vi "HEWH RLT PRAT.vi"() -> ()   [LabVIEW 2023] (continued)
            w3292 = 42 items=["No error", "Argument error", "Memory is full", "Out of zone", "End of file", "File already open", "Generic file I/O error", "File not found", "File permission error", "Disk is full", "Duplicate path", "Too many files open", "System feature not enabled", "Resource file not found", "Cannot add resource", "Resource not found", "Image not found", "Image memory error", "Pen does not exist", "Config type invalid", "Config token not found", "Config parse error", "Config memory error", "Bad external code format", "Bad external code offset", "External code not present", "Null window", "Destroy window error", "Null menu", "Print aborted", "Bad print record", "Print driver error", "Windows error during printing", "Memory error during printing", "Print dialog error", "Generic print error", "Invalid device refnum", "Device not found", "Device parameter error", "Device unit error", "Cannot open device", "Device call aborted", "Generic error", "Cancelled by user", "Object ID too low", "Object ID too high", "Object not in heap", "Unknown heap", "Unknown object (invalid DefProc)", "Unknown object (DefProc not in table)", "Message out of range", "Invalid (null) method", "Unknown message", "Manager call not supported", "Bad address", "Network operation in progress", "Network operation timed out", "Connection is busy", "Network attribute not supported", "Network error", "Address in use", "System out of memory", "Connection aborted", "Connection refused", "Not connected", "Already connected", "Connection closed", "Initialization error (interapplication manager)", "Bad occurrence", "Wait on unbound occurrence handler", "Occurrence queue overflow", "Datalog type conflict", "Unused", "Unrecognized type (interapplication manager)", "Memory corrupt", "Failed to make temporary DLL", "Old CIN version", "Drag socket not found", "Failed to load drop-object", "Failed to register OLE object", "Failed to release OLE object", "Format specifier type mismatch", "Unknown format specifier", "Too few format specifiers", "Too many format specifiers", "Scan failed", "Newer CIN version", "Error converting to variant", "Runtime menu error", "Password tampered", "Variant attribute not found", "Incompatible variant data type", "Event data is not available", "Event Store is not present", "Occurrence is not found", "Event Queue is not created", "Event info is not available", "Refnum passed is NULL", "Error retrieving Class GUID", "Error retrieving CoClass GUID", "Error retrieving TypeLib GUID.", "Bad built application magic bytes.", "Specific driver is different from the specific driver associated with the Logical Name.", "There is no session opened to the class driver.", "Max Error", "MAX - Error with config objects", "MAX - Error loading configuration", "MAX - Group not supported"]
            # "Current State"
            # "Handle mistyped state name (developer tool)"
            n1346 = Format Into String(format string="Software Exception: Unhandled State \"%s\"." ("message"), error in=w3288, w3283) -> (resulting string=w3291:string, error out=w3290:errorcluster)  [unwired: 1 in]
            n1347 = call <vilib>:"Error Cluster From Error Code.vi"("show call chain? (False)"=TRUE, "error in (no error)"=w3290, "error message (\"\")"=w3291, "error code (0)"=w3292) -> ("error out"=w3289:errorcluster)  [unwired: 5 in]
            n1348 = call <vilib>:"Add State(s) to Queue__jki_lib_state_machine.vi"("State(s) in (\"\")"=w3287) -> ("States Out"=w3286:string)  [unwired: 14 in]
          }
          frame "Error Handler" {
            # "Unhandled Error -- Display it"
            # "Clear error"
            n1349 = call <vilib>:"General Error Handler.vi"("error in (no error)"=w3295) -> ()  [unwired: 10 in, 5 out]
            n1350 = call <vilib>:"Add State(s) to Queue__jki_lib_state_machine.vi"("State(s) in Front (\"\")"="/* Post Error States", "State(s) in (\"\")"=w3299) -> ("States Out"=w3298:string)  [unwired: 13 in]
          }
          frame "Exit" {
            n1351 = call <vilib>:"Add State(s) to Queue__jki_lib_state_machine.vi"("State(s) in (\"\")"=w3304) -> ("States Out"=w3303:string)  [unwired: 14 in]
          }
          frame "---------- Data ----------" {
            n1352 = call <vilib>:"Add State(s) to Queue__jki_lib_state_machine.vi"("State(s) in (\"\")"=w3308) -> ("States Out"=w3307:string)  [unwired: 14 in]
          }
          frame "Data: Initialize" {
            n1353 = Wait on Notification(notifier=w3309, error in (no error)=w3311) -> (error out=w3310:errorcluster)  [unwired: 2 in, 3 out]
            n1354 = call "Simple Splash Screen 2012 NIVerified.vi"("Start Splash Screen"=TRUE, "error in (no error)"=w3310) -> ("error out"=w3313:errorcluster)  [unwired: 9 in]
            n1355 = while {
              tunnel: [w3337] -> w3323
              tunnel: ["User Controls"] -> w3322
              tunnel: [w3327] -> w3321
              tunnel: [w3336] -> w3320
              tunnel: [w3334] -> w3319
              tunnel: [w3333] -> w3317
              tunnel: [w3332] -> w3316
              tunnel: [w3331] -> w3315
              tunnel: [w3326] -> w3314
              tunnel: w3313 -> [w3326]
              stop <- w3328 stop-if-true
              w3332 = i16 0  # MIX VALVE STEP OFFSET
              w3333 = dbl[][] []  # Cal Build Array
              w3336 = T102 {"EEV Over A"=FALSE, "EEV Over B"=FALSE, "EEV Over C"=FALSE, "EEV Over D"=FALSE, "T-Out Over A"=FALSE, "T-Out Over B"=FALSE, "T-Out Over C"=FALSE, "T-Out Over D"=FALSE}  # Alarms
              w3337 = T95 {"Current VI Reference"=refnum, "Close Panel on Exit?"=FALSE}  # Core
              # "I use this a a temporary array to build\nall of the cal data"
              n1356 = local read "Init Complete"() -> (w3329:bool)
              n1357 = local read "DAQ Complete"() -> (w3330:bool)
              n1358 = Wait Until Next ms Multiple(millisecond multiple=u32 250) -> ()  [unwired: 1 out]
              n1359 = local read "Test Fixture Hardware Draw Loop"() -> (w3327:T55)
              n1360 = And(x=w3329, y=w3330) -> (x .and. y?=w3328:bool)
              n1361 = local read "Core HEWH Data Input A"() -> (w3331:T13)
              n1362 = local read "LV Program"() -> (w3334:T25)
            }
            n1363 = call <vilib>:"Add State(s) to Queue__jki_lib_state_machine.vi"("State(s) in (\"\")"=w3325) -> ("States Out"=w3324:string)  [unwired: 14 in]
            n1364 = Bundle("Core"=w3323, "User Controls"=w3322, "Test Fixture Hardware Draw Loop"=w3321, "Alarms"=w3320, "LV Program"=w3319, "Cal Build Array"=w3317, "MIX VALVE STEP OFFSET"=w3316, "Core HEWH Data Input A"=w3315) -> (w3318:T103)  [unwired: 1 in]
          }
          frame "---------- Valve Control ----------" {
            n1365 = call <vilib>:"Add State(s) to Queue__jki_lib_state_machine.vi"("State(s) in (\"\")"=w3342) -> ("States Out"=w3341:string)  [unwired: 14 in]
          }
          frame "Start Shutdown" {
            n1366 = call <vilib>:"Add State(s) to Queue__jki_lib_state_machine.vi"("State(s) in (\"\")"=w3347) -> ("States Out"=w3346:string)  [unwired: 14 in]
            "Shutdown" <- "Macro: Exit"
          }
          frame "Mix Valve Step Control" {
            n1367 = local read item#-1() -> (w3353)
            n1368 = case shown="\"A\"" w3353 {
              tunnel: w3352 -> [w3357 w3366]
              tunnel: [w3357 w3365] -> w3351
              tunnel: w3350 -> [w3356 w3361]
              tunnel: w3349 -> [_ w3367]
              tunnel: [w3356 w3360] -> w3348
              frame "", Default {
              }
              frame "A" {
                n1369 = Unbundle By Name(w3361) -> ("Test Fixture Hardware Draw Loop"=w3371:T55, "User Controls.Proportional Valve"=w3362:dbl)
                n1370 = call "PROPORTIONING VALVE MicroAmp Set.vi"("Refnum in"=w3367, "milliseconds to wait"=u32 100, "Debug"=FALSE, "Use Micro Amp Set"=FALSE, "error in (no error)"=w3366, "Target"=w3362, "Test Fixture Hardware"=w3371) -> ("error out"=w3365:errorcluster)  [unwired: 3 in, 1 out]
                n1371 = Greater?(x=w3362, y="Proportioning Valve Upper Limit") -> (0:w3363:bool)
                n1372 = case shown="True" w3363 {
                  tunnel: w3362 -> [w3374 w3378]
                  tunnel: [w3373 w3376] -> w3359
                  tunnel: "Auto Step Increment" -> [w3372 w3377]
                  frame False {
                    n1373 = Add(x=w3372, y=w3374) -> (x+y=w3373:dbl)
                  }
                  frame True {
                    n1374 = local write "Proportioning Valve Upper Limit"(0.0 ("Proportioning Valve Upper Limit")) -> ()
                    n1375 = Subtract(x=w3378, y=w3377) -> (x-y=w3376:dbl)
                  }
                }
                n1376 = local write "Proportioning\nValve"(w3359) -> ()
                n1377 = Bundle By Name(cluster=w3361, "User Controls.Proportional Valve"=w3359) -> (w3360:T103)
              }
            }
            n1378 = call <vilib>:"Add State(s) to Queue__jki_lib_state_machine.vi"("State(s) in (\"\")"=w3355) -> ("States Out"=w3354:string)  [unwired: 14 in]
          }
          frame "--------Intellifaucet Control------" {
            n1379 = call <vilib>:"Add State(s) to Queue__jki_lib_state_machine.vi"("State(s) in (\"\")"=w3382) -> ("States Out"=w3381:string)  [unwired: 14 in]
          }
          frame "---------ANSI Rate Test--------" {
          }
          frame "Get Rates" {
            # "Need to clean this up. Reduce number of variables in multiple locations"
            n1380 = call "HEWH HHV Notifier.vi"("Status"=UTILITY_Notifier."Read", "error in (no error)"=w3389, "name (unnamed)"="HHVData") -> ("error out"=w3388:errorcluster, "Gas Measurment Data Output"=w3387:T53)  [unwired: 7 in]
            n1381 = Unbundle By Name(w3387) -> ("Gross Heating Value, Vol (Real, Dry)"=w3386:dbl)
            n1382 = local read "Software Elapsed Time"() -> (w3402:T29)
            n1383 = local read "Gas Measurment Data"() -> (w3398:T65)
            n1384 = local read "CO CO2 Data Array"() -> (w3393:string[][])
            n1385 = Unbundle By Name(w3401) -> ("Core HEWH Data Input A.ANSI Rate"=w3400:T27)
            n1386 = call "HEWH Get Rates.vi"("Software Elapsed Time"=w3402, "Test Type - Rate"="Test Type - Rate", "ANSI Rate in"=w3400, "Gas Measurment Data"=w3398, "error in (no error)"=w3388, "Gross Heating Value, Vol (Real, Dry)"=w3386, "CO CO2 Data Array"=w3393) -> ("ANSI Display 1"=→"ANSI Display 1":string, "Rate Outputs"=→"Rate Outputs":string[][], "Test Complete"=w3395:bool, "ANSI Rate out"=w3399:T27, "Raw Timer Output"=→"Raw Timer Output":T29, "error out"=w3403:errorcluster)  [unwired: 3 in]
            n1387 = case shown="True" w3395 {
              frame False {
              }
              frame True {
                n1388 = property on="Start ANSI UI" class="Bool (strict)"("Value"=FALSE ("Start ANSI UI")) -> ()  [unwired: 2 in, 2 out]
              }
            }
            n1389 = Bundle By Name(cluster=w3401, "Core HEWH Data Input A.ANSI Rate"=w3399) -> (w3404:T103)
          }
        }
      }
    }
    frame Enabled {
    }
  }
  n1390 = Merge Errors(w70, w31) -> (w69:errorcluster)
  n1391 = Unbundle By Name(w32) -> ("WT300"=w43:refnum<queue>, "Laurel"=w45:refnum<queue>, "Emerson"=w48:refnum<queue>, "Ritter GasMeter"=w49:refnum<queue>, "Alicat_GasMeter"=w55:refnum<queue>, "Viasala Humidity"=w76:refnum<queue>, "Tenney Chamber"=w72:refnum<queue>, "UI"=w59:refnum<queue>, "GEA3-Station A"=w40:refnum<queue>, "GEA3-Station B"=w22:refnum<queue>, "GEA3-Station C"=w21:refnum<queue>, "GEA3-Station D"=w20:refnum<queue>, "MW100"=w35:refnum<queue>, "Timer"=w29:refnum<queue>, "Inficon_NG"=w28:refnum<queue>, "Inficon_LP"=w27:refnum<queue>, "Ultramat 23"=w26:refnum<queue>, "VestaCom"=w25:refnum<queue>, "EnviraCom"=w24:refnum<queue>, "Ultramat 23"=w23:refnum<queue>, "Heise Barometer"=w19:refnum<queue>, "34972A"=w18:refnum<queue>)
  n1392 = while {
    tunnel: w59 -> [w3413]
    shift-right: [w3411] -> w63
    shift-left: w67 -> [w3412]
    tunnel: [w3407] -> w66
    stop <- w3409 stop-if-true
    # "Event Handling Loop"
    n1393 = event shown="[62] \"Manual Heating Value\": Value Change" {
      selector: w3412 -> [_ _ _ _ _ _ _ _ _ _ _ _ _ _ _ _ _ _ _ _ _ _ _ _ _ _ _ _ _ _ _ _ _ _ _ _ _ _ _ _ _ _ _ _ _ _ _ _ _ _ _ _ _ _ _ _ _ _ _ _ _ _ _ _ _ _ _ _ _ _ _ _ _ _ _ _ _ _ _ _ _ _ _ _ _ _ _]
      dyn-events: [_ _ _ _ _ _ _ _ _ _ _ _ _ _ _ _ _ _ _ _ _ _ _ _ _ _ _ _ _ _ _ _ _ _ _ _ _ _ _ _ _ _ _ _ _ _ _ _ _ _ _ _ _ _ _ _ _ _ _ _ _ _ _ _ _ _ _ _ _ _ _ _ _ _ _ _ _ _ _ _ _ _ _ _ _ _ _] -> w3411
      timeout: _ -> [_ _ _ _ _ _ _ _ _ _ _ _ _ _ _ _ _ _ _ _ _ _ _ _ _ _ _ _ _ _ _ _ _ _ _ _ _ _ _ _ _ _ _ _ _ _ _ _ _ _ _ _ _ _ _ _ _ _ _ _ _ _ _ _ _ _ _ _ _ _ _ _ _ _ _ _ _ _ _ _ _ _ _ _ _ _ _]
      tunnel: [TRUE ("Discard?") _ _ _ _ _ _ _ _ _ _ _ _ _ _ _ _ _ _ _ _ _ _ _ _ _ _ _ _ _ _ _ _ _ _ _ _ _ _ _ _ _ _ _ _ _ _ _ _ _ _ _ _ _ _ _ _ _ _ _ _ _ _ _ _ _ _ _ _ _ _ _ _ _ _ _ _ _ _ _ _ _ _ _ _ _ _] -> w3409
      tunnel: w3413 -> [w3415 w3416 w3422 w3429 w3433 w3443 w3453 w3463 w3474 w3476 w3485 w3491 w3497 w3503 w3504 w3509 w3514 w3519 w3526 w3531 w3536 w3542 w3547 w3552 w3557 w3562 w3567 w3572 w3577 w3582 w3587 w3592 w3597 w3602 w3607 w3612 w3617 w3622 w3627 w3632 w3637 w3642 w3647 w3652 w3659 w3664 w3669 w3674 w3679 w3684 w3689 w3694 w3700 w3706 w3712 w3715 w3720 w3725 w3730 w3733 w3738 w3743 w3749 w3755 w3761 w3768 w3775 w3784 w3791 w3798 w3805 w3812 w3819 w3826 w3833 w3839 w3845 w3851 w3857 w3863 w3869 w3875 w3880 w3886 w3892 w3898 w3906]
      tunnel: [_ _ w3421 w3428 w3431 w3441 w3451 w3461 w3471 w3477 w3482 w3488 w3494 w3500 w3506 w3511 w3516 w3521 w3524 w3529 w3534 w3540 w3545 w3550 w3555 w3560 w3565 w3570 w3575 w3580 w3585 w3590 w3595 w3600 w3605 w3610 w3615 w3620 w3625 w3630 w3635 w3640 w3645 w3650 w3656 w3661 w3666 w3671 w3676 w3681 w3686 w3691 w3697 w3703 w3709 w3713 w3718 w3723 w3728 w3735 w3740 w3745 w3751 w3757 w3763 _ w3773 w3782 w3789 w3796 w3803 w3810 w3817 w3824 w3831 w3837 w3843 w3849 w3855 w3861 w3867 w3873 w3881 w3887 w3893 w3899 w3904] -> w3410
      tunnel: [w3415 w3416 w3420 w3427 w3432 w3442 w3452 w3462 w3473 w3475 w3484 w3490 w3496 w3502 w3505 w3510 w3515 w3520 w3525 w3530 w3535 w3541 w3546 w3551 w3556 w3561 w3566 w3571 w3576 w3581 w3586 w3591 w3596 w3601 w3606 w3611 w3616 w3621 w3626 w3631 w3636 w3641 w3646 w3651 w3658 w3663 w3668 w3673 w3678 w3683 w3688 w3693 w3699 w3705 w3711 w3714 w3719 w3724 w3729 w3734 w3739 w3744 w3750 w3756 w3762 w3767 w3774 w3783 w3790 w3797 w3804 w3811 w3818 w3825 w3832 w3838 w3844 w3850 w3856 w3862 w3868 w3874 w3878 w3884 w3890 w3896 w3905] -> w3408
      event User Event {
        # "The Message Handling Loop processed an \"Exit\" message, which fired this event to stop the Event Handling Loop."
        n1394 = event-data() -> ()  [unwired: 1 in, 1 out]
      }
      event Application Instance Close {
        # "#CodeRecommended - When a project closes, all VIs within that project are aborted and leave memory. However, any code placed in this event frame is guaranteed to run to completion, so add any cleanup code that absolutely must happen here."
        n1395 = event-data() -> ()  [unwired: 1 in, 1 out]
      }
      event Panel Close? {
        n1396 = event-data() -> ()  [unwired: 1 in, 1 out]
        n1397 = Stop(stop? (T)=TRUE) -> ()
        n1398 = call-poly "Enqueue Message.vi"("Priority Message? (F)"=TRUE, "Message"="Exit", "Message Queue"=w3422) -> ("error out"=w3421:errorcluster, "dup Message Queue"=w3420:refnum<queue>)  [unwired: 7 in]
        n1399 = event-data("Discard?"=TRUE) -> ()  [unwired: 1 in, 1 out]
      }
      event "Finish": Value Change {
        n1400 = event-data() -> ()  [unwired: 1 in, 1 out]
        n1401 = call-poly "Enqueue Message.vi"("Priority Message? (F)"=TRUE, "Message"="Exit", "Message Queue"=w3429) -> ("error out"=w3428:errorcluster, "dup Message Queue"=w3427:refnum<queue>)  [unwired: 7 in]
        n1402 = Stop(stop? (T)=TRUE) -> ()
      }
      event "Reset Timer (A)": Value Change {
        n1403 = event-data() -> ("NewVal"=w3430:bool)  [unwired: 1 in]
        n1404 = case shown="True" w3430 {
          tunnel: w3433 -> [w3434 w3439]
          tunnel: [w3434 w3438] -> w3432
          tunnel: [_ w3436] -> w3431
          frame False {
          }
          frame True {
            n1405 = call-poly "Enqueue Message.vi"("Priority Message? (F)"=TRUE, "Message"="Reset_TimerA_UI", "Message Queue"=w3439) -> ("error out"=w3436:errorcluster, "dup Message Queue"=w3438:refnum<queue>)  [unwired: 7 in]
          }
        }
      }
      event "Reset Timer (B)": Value Change {
        n1406 = event-data() -> ("NewVal"=w3440:bool)  [unwired: 1 in]
        n1407 = case shown="True" w3440 {
          tunnel: w3443 -> [w3444 w3449]
          tunnel: [w3444 w3448] -> w3442
          tunnel: [_ w3446] -> w3441
          frame False {
          }
          frame True {
            n1408 = call-poly "Enqueue Message.vi"("Priority Message? (F)"=TRUE, "Message"="Reset_TimerB_UI", "Message Queue"=w3449) -> ("error out"=w3446:errorcluster, "dup Message Queue"=w3448:refnum<queue>)  [unwired: 7 in]
          }
        }
      }
      event "Reset Timer (C)": Value Change {
        n1409 = event-data() -> ("NewVal"=w3450:bool)  [unwired: 1 in]
        n1410 = case shown="True" w3450 {
          tunnel: w3453 -> [w3454 w3459]
          tunnel: [w3454 w3458] -> w3452
          tunnel: [_ w3456] -> w3451
          frame False {
          }
          frame True {
            n1411 = call-poly "Enqueue Message.vi"("Priority Message? (F)"=TRUE, "Message"="Reset_TimerC_UI", "Message Queue"=w3459) -> ("error out"=w3456:errorcluster, "dup Message Queue"=w3458:refnum<queue>)  [unwired: 7 in]
          }
        }
      }
      event "Reset Timer (D)": Value Change {
        n1412 = event-data() -> ("NewVal"=w3460:bool)  [unwired: 1 in]
        n1413 = case shown="False" w3460 {
          tunnel: w3463 -> [w3464 w3469]
          tunnel: [w3464 w3468] -> w3462
          tunnel: [_ w3466] -> w3461
          frame False {
          }
          frame True {
            n1414 = call-poly "Enqueue Message.vi"("Priority Message? (F)"=TRUE, "Message"="Reset_TimerD_UI", "Message Queue"=w3469) -> ("error out"=w3466:errorcluster, "dup Message Queue"=w3468:refnum<queue>)  [unwired: 7 in]
          }
        }
      }
      event "Set Temperature": Value Change {
        n1415 = event-data() -> ()  [unwired: 1 in, 1 out]
        n1416 = call-poly "Enqueue Message.vi"("Priority Message? (F)"=TRUE, "Message"="PUT_Tenney_Temp_UI", "Message Queue"=w3474) -> ("error out"=w3471:errorcluster, "dup Message Queue"=w3473:refnum<queue>)  [unwired: 7 in]
      }
      event "Cancel Draw": Value Change {
        n1417 = event-data() -> ()  [unwired: 1 in, 1 out]
        n1418 = call-poly "Enqueue Message.vi"("Priority Message? (F)"=TRUE, "Message"="Cancel_Draw_UI", "Message Queue"=w3476) -> ("error out"=w3477:errorcluster, "dup Message Queue"=w3475:refnum<queue>)  [unwired: 7 in]
      }
      event "DAQ for A": Value Change {
        n1419 = event-data() -> ("NewVal"=w3480:bool)  [unwired: 1 in]
        n1420 = call-poly "Enqueue Message.vi"("Priority Message? (F)"=TRUE, "Message Data"=w3480, "Message"="DAQ_for_A_UI", "Message Queue"=w3485) -> ("error out"=w3482:errorcluster, "dup Message Queue"=w3484:refnum<queue>)  [unwired: 6 in]
      }
      event "DAQ for B": Value Change {
        n1421 = event-data() -> ("NewVal"=w3486:bool)  [unwired: 1 in]
        n1422 = call-poly "Enqueue Message.vi"("Priority Message? (F)"=TRUE, "Message Data"=w3486, "Message"="DAQ_for_B_UI", "Message Queue"=w3491) -> ("error out"=w3488:errorcluster, "dup Message Queue"=w3490:refnum<queue>)  [unwired: 6 in]
      }
      event "DAQ for C": Value Change {
        n1423 = event-data() -> ("NewVal"=w3492:bool)  [unwired: 1 in]
        n1424 = call-poly "Enqueue Message.vi"("Priority Message? (F)"=TRUE, "Message Data"=w3492, "Message"="DAQ_for_C_UI", "Message Queue"=w3497) -> ("error out"=w3494:errorcluster, "dup Message Queue"=w3496:refnum<queue>)  [unwired: 6 in]
      }
      event "DAQ for D": Value Change {
        n1425 = event-data() -> ("NewVal"=w3498:bool)  [unwired: 1 in]
        n1426 = call-poly "Enqueue Message.vi"("Priority Message? (F)"=TRUE, "Message Data"=w3498, "Message"="DAQ_for_D_UI", "Message Queue"=w3503) -> ("error out"=w3500:errorcluster, "dup Message Queue"=w3502:refnum<queue>)  [unwired: 6 in]
      }
      event "X-Axis - Station A", "Y-Axis1 - Station A", "Y-Axis2 - Station A": Value Change {
        n1427 = event-data() -> ()  [unwired: 1 in, 1 out]
        n1428 = call-poly "Enqueue Message.vi"("Priority Message? (F)"=TRUE, "Message"="Update_Graph_StationA_UI", "Message Queue"=w3504) -> ("error out"=w3506:errorcluster, "dup Message Queue"=w3505:refnum<queue>)  [unwired: 7 in]
      }
      event "X-Axis - Station B", "Y-Axis1 - Station B", "Y-Axis2 - Station B": Value Change {
        n1429 = event-data() -> ()  [unwired: 1 in, 1 out]
        n1430 = call-poly "Enqueue Message.vi"("Priority Message? (F)"=TRUE, "Message"="Update_Graph_StationB_UI", "Message Queue"=w3509) -> ("error out"=w3511:errorcluster, "dup Message Queue"=w3510:refnum<queue>)  [unwired: 7 in]
      }
      event "X-Axis - Station C", "Y-Axis1 - Station C", "Y-Axis2 - Station C": Value Change {
        n1431 = event-data() -> ()  [unwired: 1 in, 1 out]
        n1432 = call-poly "Enqueue Message.vi"("Priority Message? (F)"=TRUE, "Message"="Update_Graph_StationC_UI", "Message Queue"=w3514) -> ("error out"=w3516:errorcluster, "dup Message Queue"=w3515:refnum<queue>)  [unwired: 7 in]
      }
      event "X-Axis - Station D", "Y-Axis1 - Station D", "Y-Axis2 - Station D": Value Change {
        n1433 = event-data() -> ()  [unwired: 1 in, 1 out]
        n1434 = call-poly "Enqueue Message.vi"("Priority Message? (F)"=TRUE, "Message"="Update_Graph_StationD_UI", "Message Queue"=w3519) -> ("error out"=w3521:errorcluster, "dup Message Queue"=w3520:refnum<queue>)  [unwired: 7 in]
      }
      event "Enable EMV ERD List": Value Change {
        n1435 = event-data() -> ()  [unwired: 1 in, 1 out]
        n1436 = call-poly "Enqueue Message.vi"("Priority Message? (F)"=TRUE, "Message"="Enable_EMV_List_StationA_UI", "Message Queue"=w3526) -> ("error out"=w3524:errorcluster, "dup Message Queue"=w3525:refnum<queue>)  [unwired: 7 in]
      }
      event "Enable Inverter ERD List": Value Change {
        n1437 = event-data() -> ()  [unwired: 1 in, 1 out]
        n1438 = call-poly "Enqueue Message.vi"("Priority Message? (F)"=TRUE, "Message"="Enable_Inverter_List_StationA_UI", "Message Queue"=w3531) -> ("error out"=w3529:errorcluster, "dup Message Queue"=w3530:refnum<queue>)  [unwired: 7 in]
      }
      event "Enable Heat Pump ERD List": Value Change {
        n1439 = event-data() -> ()  [unwired: 1 in, 1 out]
        n1440 = call-poly "Enqueue Message.vi"("Priority Message? (F)"=TRUE, "Message"="Enable_HeatPump_List_StationA_UI", "Message Queue"=w3536) -> ("error out"=w3534:errorcluster, "dup Message Queue"=w3535:refnum<queue>)  [unwired: 7 in]
      }
      event "GEA2_A?", "GEA2_B?", "GEA2_C?", "GEA2_D?": Value Change {
        n1441 = event-data() -> ("NewVal"=w3539:bool)  [unwired: 1 in]
        n1442 = call-poly "Enqueue Message.vi"("Priority Message? (F)"=TRUE, "Message Data"=w3539, "Message"="GEA3_Controls_UI", "Message Queue"=w3542) -> ("error out"=w3540:errorcluster, "dup Message Queue"=w3541:refnum<queue>)  [unwired: 6 in]
      }
      event Value Change {
        n1443 = event-data() -> ()  [unwired: 1 in, 1 out]
        n1444 = call-poly "Enqueue Message.vi"("Priority Message? (F)"=TRUE, "Message"="Inlet_Valve_A_MW100_UI", "Message Queue"=w3547) -> ("error out"=w3545:errorcluster, "dup Message Queue"=w3546:refnum<queue>)  [unwired: 7 in]
      }
      event Value Change {
        n1445 = event-data() -> ()  [unwired: 1 in, 1 out]
        n1446 = call-poly "Enqueue Message.vi"("Priority Message? (F)"=TRUE, "Message"="Inlet_Valve_B_MW100_UI", "Message Queue"=w3552) -> ("error out"=w3550:errorcluster, "dup Message Queue"=w3551:refnum<queue>)  [unwired: 7 in]
      }
      event Value Change {
        n1447 = event-data() -> ()  [unwired: 1 in, 1 out]
        n1448 = call-poly "Enqueue Message.vi"("Priority Message? (F)"=TRUE, "Message"="Inlet_Valve_C_MW100_UI", "Message Queue"=w3557) -> ("error out"=w3555:errorcluster, "dup Message Queue"=w3556:refnum<queue>)  [unwired: 7 in]
      }
      event Value Change {
        n1449 = event-data() -> ()  [unwired: 1 in, 1 out]
        n1450 = call-poly "Enqueue Message.vi"("Priority Message? (F)"=TRUE, "Message"="Inlet_Valve_D_MW100_UI", "Message Queue"=w3562) -> ("error out"=w3560:errorcluster, "dup Message Queue"=w3561:refnum<queue>)  [unwired: 7 in]
      }
      event Value Change {
        n1451 = event-data() -> ()  [unwired: 1 in, 1 out]
        n1452 = call-poly "Enqueue Message.vi"("Priority Message? (F)"=TRUE, "Message"="Drain_Valve_A_MW100_UI", "Message Queue"=w3567) -> ("error out"=w3565:errorcluster, "dup Message Queue"=w3566:refnum<queue>)  [unwired: 7 in]
      }
      event Value Change {
        n1453 = event-data() -> ()  [unwired: 1 in, 1 out]
        n1454 = call-poly "Enqueue Message.vi"("Priority Message? (F)"=TRUE, "Message"="Drain_Valve_B_MW100_UI", "Message Queue"=w3572) -> ("error out"=w3570:errorcluster, "dup Message Queue"=w3571:refnum<queue>)  [unwired: 7 in]
      }
      event Value Change {
        n1455 = event-data() -> ()  [unwired: 1 in, 1 out]
        n1456 = call-poly "Enqueue Message.vi"("Priority Message? (F)"=TRUE, "Message"="Drain_Valve_C_MW100_UI", "Message Queue"=w3577) -> ("error out"=w3575:errorcluster, "dup Message Queue"=w3576:refnum<queue>)  [unwired: 7 in]
      }
      event Value Change {
        n1457 = event-data() -> ()  [unwired: 1 in, 1 out]
        n1458 = call-poly "Enqueue Message.vi"("Priority Message? (F)"=TRUE, "Message"="Drain_Valve_D_MW100_UI", "Message Queue"=w3582) -> ("error out"=w3580:errorcluster, "dup Message Queue"=w3581:refnum<queue>)  [unwired: 7 in]
      }
      event Value Change {
        n1459 = event-data() -> ()  [unwired: 1 in, 1 out]
        n1460 = call-poly "Enqueue Message.vi"("Priority Message? (F)"=TRUE, "Message"="Outlet_Valve_A_MW100_UI", "Message Queue"=w3587) -> ("error out"=w3585:errorcluster, "dup Message Queue"=w3586:refnum<queue>)  [unwired: 7 in]
      }
      event Value Change {
        n1461 = event-data() -> ()  [unwired: 1 in, 1 out]
        n1462 = call-poly "Enqueue Message.vi"("Priority Message? (F)"=TRUE, "Message"="Outlet_Valve_B_MW100_UI", "Message Queue"=w3592) -> ("error out"=w3590:errorcluster, "dup Message Queue"=w3591:refnum<queue>)  [unwired: 7 in]
      }
      event Value Change {
        n1463 = event-data() -> ()  [unwired: 1 in, 1 out]
        n1464 = call-poly "Enqueue Message.vi"("Priority Message? (F)"=TRUE, "Message"="Outlet_Valve_C_MW100_UI", "Message Queue"=w3597) -> ("error out"=w3595:errorcluster, "dup Message Queue"=w3596:refnum<queue>)  [unwired: 7 in]
      }
      event Value Change {
        n1465 = event-data() -> ()  [unwired: 1 in, 1 out]
        n1466 = call-poly "Enqueue Message.vi"("Priority Message? (F)"=TRUE, "Message"="Outlet_Valve_D_MW100_UI", "Message Queue"=w3602) -> ("error out"=w3600:errorcluster, "dup Message Queue"=w3601:refnum<queue>)  [unwired: 7 in]
      }
      event "Set Valves-A": Value Change {
        n1467 = event-data() -> ()  [unwired: 1 in, 1 out]
        n1468 = call-poly "Enqueue Message.vi"("Priority Message? (F)"=TRUE, "Message"="Set_Valves_StationA_MW100_UI", "Message Queue"=w3607) -> ("error out"=w3605:errorcluster, "dup Message Queue"=w3606:refnum<queue>)  [unwired: 7 in]
      }
      event "Set Valves-B": Value Change {
        n1469 = event-data() -> ()  [unwired: 1 in, 1 out]
        n1470 = call-poly "Enqueue Message.vi"("Priority Message? (F)"=TRUE, "Message"="Set_Valves_StationB_MW100_UI", "Message Queue"=w3612) -> ("error out"=w3610:errorcluster, "dup Message Queue"=w3611:refnum<queue>)  [unwired: 7 in]
      }
      event "Set Valves-C": Value Change {
        n1471 = event-data() -> ()  [unwired: 1 in, 1 out]
        n1472 = call-poly "Enqueue Message.vi"("Priority Message? (F)"=TRUE, "Message"="Set_Valves_StationC_MW100_UI", "Message Queue"=w3617) -> ("error out"=w3615:errorcluster, "dup Message Queue"=w3616:refnum<queue>)  [unwired: 7 in]
      }
      event "Set Valves-D": Value Change {
        n1473 = event-data() -> ()  [unwired: 1 in, 1 out]
        n1474 = call-poly "Enqueue Message.vi"("Priority Message? (F)"=TRUE, "Message"="Set_Valves_StationD_MW100_UI", "Message Queue"=w3622) -> ("error out"=w3620:errorcluster, "dup Message Queue"=w3621:refnum<queue>)  [unwired: 7 in]
      }
      event "Main Power": Value Change {
        n1475 = event-data() -> ()  [unwired: 1 in, 1 out]
        n1476 = call-poly "Enqueue Message.vi"("Priority Message? (F)"=TRUE, "Message"="MainPower_MW100_UI", "Message Queue"=w3627) -> ("error out"=w3625:errorcluster, "dup Message Queue"=w3626:refnum<queue>)  [unwired: 7 in]
      }
      event "IF Start": Value Change {
        n1477 = event-data() -> ()  [unwired: 1 in, 1 out]
        n1478 = call-poly "Enqueue Message.vi"("Priority Message? (F)"=TRUE, "Message"="Start_Intellifaucet_MW100_UI", "Message Queue"=w3632) -> ("error out"=w3630:errorcluster, "dup Message Queue"=w3631:refnum<queue>)  [unwired: 7 in]
      }
      event "IF Stop": Value Change {
        n1479 = event-data() -> ()  [unwired: 1 in, 1 out]
        n1480 = call-poly "Enqueue Message.vi"("Priority Message? (F)"=TRUE, "Message"="Stop_Intellifaucet_MW100_UI", "Message Queue"=w3637) -> ("error out"=w3635:errorcluster, "dup Message Queue"=w3636:refnum<queue>)  [unwired: 7 in]
      }
      event "Temp (°F)": Value Change {
        n1481 = event-data() -> ()  [unwired: 1 in, 1 out]
        n1482 = call-poly "Enqueue Message.vi"("Priority Message? (F)"=TRUE, "Message"="Adjust_Temp_Intellifaucet_MW100_UI", "Message Queue"=w3642) -> ("error out"=w3640:errorcluster, "dup Message Queue"=w3641:refnum<queue>)  [unwired: 7 in]
      }
      event "Valve % Open": Value Change {
        n1483 = event-data() -> ()  [unwired: 1 in, 1 out]
        n1484 = call-poly "Enqueue Message.vi"("Priority Message? (F)"=TRUE, "Message"="Adjust_Flow_Intellifaucet_MW100_UI", "Message Queue"=w3647) -> ("error out"=w3645:errorcluster, "dup Message Queue"=w3646:refnum<queue>)  [unwired: 7 in]
      }
      event "Proportioning\nValve": Value Change {
        n1485 = event-data() -> ()  [unwired: 1 in, 1 out]
        n1486 = call-poly "Enqueue Message.vi"("Priority Message? (F)"=TRUE, "Message"="Adjust_Prop_Valve_MW100_UI", "Message Queue"=w3652) -> ("error out"=w3650:errorcluster, "dup Message Queue"=w3651:refnum<queue>)  [unwired: 7 in]
      }
      event "Update TankSP Offset": Value Change {
        n1487 = event-data() -> ()  [unwired: 1 in, 1 out]
        n1488 = call-poly "Enqueue Message.vi"("Priority Message? (F)"=TRUE, "Message"="Update_TankSP_Offset_StationA_UI", "Message Queue"=w3659) -> ("error out"=w3656:errorcluster, "dup Message Queue"=w3658:refnum<queue>)  [unwired: 7 in]
      }
      event "Update User Setpoint": Value Change {
        n1489 = event-data() -> ()  [unwired: 1 in, 1 out]
        n1490 = call-poly "Enqueue Message.vi"("Priority Message? (F)"=TRUE, "Message"="Update_User_Setpoint_StationA_UI", "Message Queue"=w3664) -> ("error out"=w3661:errorcluster, "dup Message Queue"=w3663:refnum<queue>)  [unwired: 7 in]
      }
      event "Update Mode": Value Change {
        n1491 = event-data() -> ()  [unwired: 1 in, 1 out]
        n1492 = call-poly "Enqueue Message.vi"("Priority Message? (F)"=TRUE, "Message"="Update_Mode_StationA_UI", "Message Queue"=w3669) -> ("error out"=w3666:errorcluster, "dup Message Queue"=w3668:refnum<queue>)  [unwired: 7 in]
      }
      event "Update Capacity": Value Change {
        n1493 = event-data() -> ()  [unwired: 1 in, 1 out]
        n1494 = call-poly "Enqueue Message.vi"("Priority Message? (F)"=TRUE, "Message"="Update_Capacity_StationA_UI", "Message Queue"=w3674) -> ("error out"=w3671:errorcluster, "dup Message Queue"=w3673:refnum<queue>)  [unwired: 7 in]
      }
      event "Update Personality": Value Change {
        n1495 = event-data() -> ()  [unwired: 1 in, 1 out]
        n1496 = call-poly "Enqueue Message.vi"("Priority Message? (F)"=TRUE, "Message"="Update_Personality_StationA_UI", "Message Queue"=w3679) -> ("error out"=w3676:errorcluster, "dup Message Queue"=w3678:refnum<queue>)  [unwired: 7 in]
      }
      event "Reset Control Counter": Value Change {
        n1497 = event-data() -> ()  [unwired: 1 in, 1 out]
        n1498 = call-poly "Enqueue Message.vi"("Priority Message? (F)"=TRUE, "Message"="Reset_Control_Counter_StationA_UI", "Message Queue"=w3684) -> ("error out"=w3681:errorcluster, "dup Message Queue"=w3683:refnum<queue>)  [unwired: 7 in]
      }
      event "Set Humidity": Value Change {
        n1499 = event-data() -> ()  [unwired: 1 in, 1 out]
        n1500 = call-poly "Enqueue Message.vi"("Priority Message? (F)"=TRUE, "Message"="PUT_Tenney_Humidity_UI", "Message Queue"=w3689) -> ("error out"=w3686:errorcluster, "dup Message Queue"=w3688:refnum<queue>)  [unwired: 7 in]
      }
      event "Set Frequency": Value Change {
        n1501 = event-data() -> ()  [unwired: 1 in, 1 out]
        n1502 = call-poly "Enqueue Message.vi"("Priority Message? (F)"=TRUE, "Message"="PUT_Tenney_Frequency_UI", "Message Queue"=w3694) -> ("error out"=w3691:errorcluster, "dup Message Queue"=w3693:refnum<queue>)  [unwired: 7 in]
      }
      event "Set Status": Value Change {
        n1503 = event-data() -> ()  [unwired: 1 in, 1 out]
        n1504 = call-poly "Enqueue Message.vi"("Priority Message? (F)"=TRUE, "Message Data"="Chamber Status", "Message"="PUT_Chamber_Status_UI", "Message Queue"=w3700) -> ("error out"=w3697:errorcluster, "dup Message Queue"=w3699:refnum<queue>)  [unwired: 6 in]
      }
      event "Enable Auto Control": Value Change {
        n1505 = event-data() -> ("NewVal"=w3702:bool)  [unwired: 1 in]
        n1506 = call-poly "Enqueue Message.vi"("Priority Message? (F)"=TRUE, "Message Data"=w3702, "Message"="Tenney_Enable_Auto_Control_UI", "Message Queue"=w3706) -> ("error out"=w3703:errorcluster, "dup Message Queue"=w3705:refnum<queue>)  [unwired: 6 in]
      }
      event "Update Temperature Limits": Value Change {
        n1507 = event-data() -> ("NewVal"=w3708:bool)  [unwired: 1 in]
        n1508 = call-poly "Enqueue Message.vi"("Priority Message? (F)"=TRUE, "Message Data"=w3708, "Message"="Update_Temp_Limits_UI", "Message Queue"=w3712) -> ("error out"=w3709:errorcluster, "dup Message Queue"=w3711:refnum<queue>)  [unwired: 6 in]
      }
      event "Sample Rate (mS)": Value Change {
        n1509 = event-data() -> ()  [unwired: 1 in, 1 out]
        n1510 = call-poly "Enqueue Message.vi"("Priority Message? (F)"=TRUE, "Message"="Set_Scan_Rate_UI", "Message Queue"=w3715) -> ("error out"=w3713:errorcluster, "dup Message Queue"=w3714:refnum<queue>)  [unwired: 7 in]
      }
      event "Reset Totalizer": Value Change {
        n1511 = event-data() -> ()  [unwired: 1 in, 1 out]
        n1512 = call-poly "Enqueue Message.vi"("Priority Message? (F)"=TRUE, "Message"="Reset_Gas_Totalizer_UI", "Message Queue"=w3720) -> ("error out"=w3718:errorcluster, "dup Message Queue"=w3719:refnum<queue>)  [unwired: 7 in]
      }
      event "Tare Meter": Value Change {
        n1513 = event-data() -> ()  [unwired: 1 in, 1 out]
        n1514 = call-poly "Enqueue Message.vi"("Priority Message? (F)"=TRUE, "Message"="Alicat_Tare_Flow_UI", "Message Queue"=w3725) -> ("error out"=w3723:errorcluster, "dup Message Queue"=w3724:refnum<queue>)  [unwired: 7 in]
      }
      event Value Change {
        n1515 = event-data() -> ()  [unwired: 1 in, 3 out]
        n1516 = call-poly "Enqueue Message.vi"("Priority Message? (F)"=TRUE, "Message"="Change_Gas_UI", "Message Queue"=w3730) -> ("error out"=w3728:errorcluster, "dup Message Queue"=w3729:refnum<queue>)  [unwired: 7 in]
      }
      event "Reset Inventory": Value Change {
        n1517 = event-data() -> ()  [unwired: 1 in, 1 out]
        n1518 = call-poly "Enqueue Message.vi"("Priority Message? (F)"=TRUE, "Message"="Reset_Inventory_Emerson_UI", "Message Queue"=w3733) -> ("error out"=w3735:errorcluster, "dup Message Queue"=w3734:refnum<queue>)  [unwired: 7 in]
      }
      event "Reset Flow Meter": Value Change {
        n1519 = event-data() -> ()  [unwired: 1 in, 1 out]
